vi "ArmGetChickenEnable.vi"() -> (0 "ChickenEnable":bool)   [LabVIEW 2020]
doc: "Getter fpr ArmChickenEnable (chicken switch)\nOutputs:\n--ChickenEnable--Boolean--"
uses:
  ArmGlobal.vi
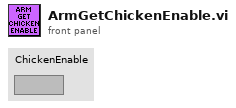
[diagram p1: front panel]
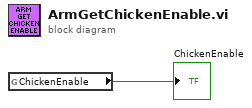
[diagram p0: block diagram]
diagram:
  n1 = global read "ArmGlobal.vi" "ChickenEnable"() -> (→"ChickenEnable":bool)
